vi "ReadWFGSettings.vi"(0 "object in":refnum<class "AD2_SDK.lvclass">, 5 "error in (no error)":errorcluster) -> (14 "object out":refnum<class "AD2_SDK.lvclass">, 16 "AmplitudeAndVoltage":T1, 19 "error out":errorcluster)   [LabVIEW 2019, in "AD2_SDK.lvclass"]
uses:
  AD2_SDK.lvclass
  AD2_WFG_SDK_class/AD2_WFG_SDK.lvclass
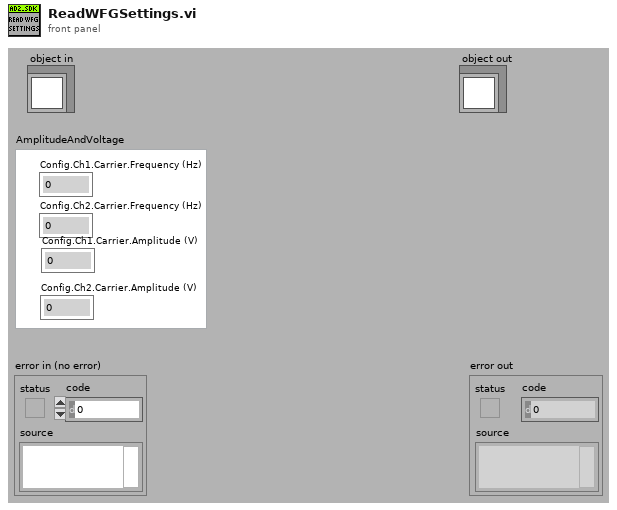
[diagram p1: front panel]
types:
  T1 = cluster{"Config.Ch1.Carrier.Frequency (Hz)":dbl, "Config.Ch2.Carrier.Frequency (Hz)":dbl, "Config.Ch1.Carrier.Amplitude (V)":dbl, "Config.Ch2.Carrier.Amplitude (V)":dbl}
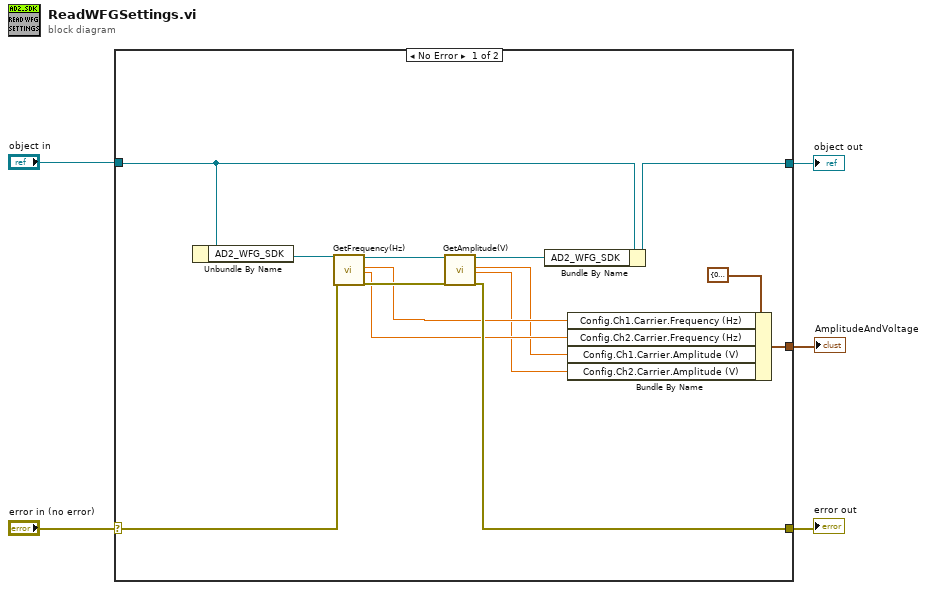
[diagram p0: block diagram]
diagram:
  n1 = case shown="No Error" "error in (no error)" {
    selector: "error in (no error)" -> [w16 w21]
    tunnel: [w12 w21] -> w4
    tunnel: [w18 w20] -> w2
    tunnel: "object in" -> [w19 w20]
    tunnel: [w6 _] -> w1
    frame No Error {
      n2 = Unbundle By Name(w19) -> ("AD2_WFG_SDK"=w17:refnum<class "AD2_WFG_SDK.lvclass">)
      n3 = call-dynamic "GetFrequency(Hz).vi"("object in"=w17, "error in (no error)"=w16) -> ("object out"=w15:refnum<class "AD2_WFG_SDK.lvclass">, "Config.Ch1.Carrier.Frequency (Hz)"=w10:dbl, "Config.Ch2.Carrier.Frequency (Hz)"=w9:dbl, "error out"=w13:errorcluster)  [unwired: 14 in]
      n4 = call-dynamic "GetAmplitude(V).vi"("object in"=w15, "error in (no error)"=w13) -> ("object out"=w14:refnum<class "AD2_WFG_SDK.lvclass">, "Config.Ch1.Carrier.Amplitude (V)"=w8:dbl, "Config.Ch2.Carrier.Amplitude (V)"=w7:dbl, "error out"=w12:errorcluster)  [unwired: 14 in]
      n5 = Bundle By Name(cluster=w19, "AD2_WFG_SDK"=w14) -> (w18:refnum<class "AD2_SDK.lvclass">)
      n6 = Bundle By Name(cluster=T1 {"Config.Ch1.Carrier.Frequency (Hz)"=0.0, "Config.Ch2.Carrier.Frequency (Hz)"=0.0, "Config.Ch1.Carrier.Amplitude (V)"=0.0, "Config.Ch2.Carrier.Amplitude (V)"=0.0} ("AmplitudeAndVoltage"), "Config.Ch1.Carrier.Frequency (Hz)"=w10, "Config.Ch2.Carrier.Frequency (Hz)"=w9, "Config.Ch1.Carrier.Amplitude (V)"=w8, "Config.Ch2.Carrier.Amplitude (V)"=w7) -> (w6:T1)
    }
    frame Error {
    }
  }
  "error out" <- w4
  "object out" <- w2
  "AmplitudeAndVoltage" <- w1
